vi "Actor Core.vi"(8 "error in (no error)":errorcluster, 11 "Test Interface in":refnum<class "Test Interface.lvclass">) -> (0 "error out":errorcluster, 3 "Actor Framework.lvlib:Actor":refnum<class "Actor.lvclass">)   [LabVIEW 2015, in "Test Interface.lvclass"]
uses:
  Test Interface.lvclass
  <vilib>/ActorFramework/Actor/Actor.lvclass
  Controls/Menu object array.ctl
  Controls/Menu object.ctl
  Test Interface.lvclass/Test Interface.ctl
  <vilib>/ActorFramework/Actor/Actor.lvclass/Actor.ctl
  <vilib>/ActorFramework/Message Enqueuer/Message Enqueuer.lvclass/Message Enqueuer.ctl
  <vilib>/ActorFramework/Message Enqueuer/Init from Existing Queue.vi
  <vilib>/ActorFramework/Message Enqueuer/Enqueue.vi
  <vilib>/ActorFramework/Message Priority Queue/Priority Enqueue.vi
  <vilib>/ActorFramework/Message Enqueuer/Message Enqueuer.lvclass
  <vilib>/ActorFramework/Stop Msg/Stop Msg.lvclass
  Mag Lab Measure Interface/Mag Lab Measure UI.lvclass
panel:
  in  "Menu object array":T1 {"Object name" items=["Select one"]}
  in  "Devices":u16[](array[ring]) items=["dev1", "5051"]
  in  "Stop Button":bool
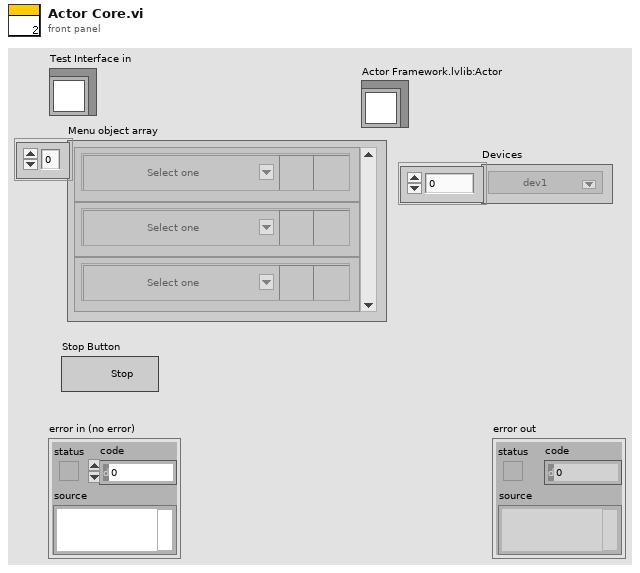
[diagram p1: front panel]
types:
  T1 = typedef "Menu object array.ctl" = T2[]
  T2 = typedef "Menu object.ctl" = cluster{"Object name":u16, "Open parameters":bool, "Remove Button":bool}
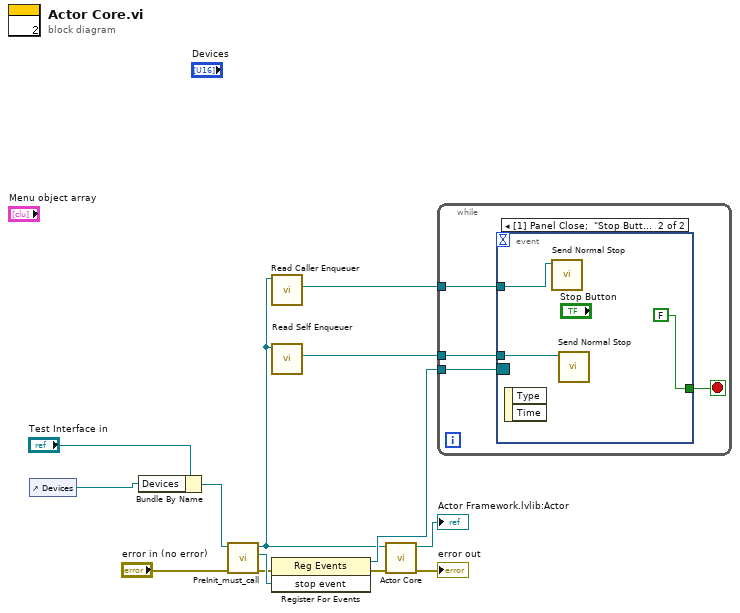
[diagram p0: block diagram]
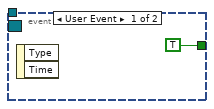
[diagram p2: hidden frame]
diagram:
  n1 = control-ref of="Devices"() -> (w1:refnum<vi>)
  n2 = Bundle By Name(cluster="Test Interface in", "Devices"=w1) -> (w2:refnum<class "Test Interface.lvclass">)
  n3 = call-dynamic "PreInit_must_call.vi"("error in (no error)"="error in (no error)", "Mag Lab Measure Interface in"=w2) -> ("error out"=w5:errorcluster, "stop event"=w11:refnum<user-event>, "Mag Lab Measure Interface out"=w4:refnum<class "Test Interface.lvclass">)  [unwired: 7 in]
  n4 = call <vilib>:"Read Caller Enqueuer.vi"("Actor"=w4) -> ("Caller Enqueuer"=w3:refnum<class "Message Enqueuer.lvclass">)  [unwired: 10 in]
  n5 = call <vilib>:"Read Self Enqueuer.vi"("Actor"=w4) -> ("Self Enqueuer"=w7:refnum<class "Message Enqueuer.lvclass">)  [unwired: 10 in]
  n6 = register-events(error in=w5, w11) -> (reference out=w8:refnum<event-registration>, error out=w9:errorcluster)  [unwired: 1 in]
  n7 = call-parent "Actor Core.vi"("error in (no error)"=w9, "Mag Lab Measure Interface in"=w4) -> ("error out"=→"error out":errorcluster, "Actor Framework.lvlib:Actor"=→"Actor Framework.lvlib:Actor":refnum<class "Actor.lvclass">)  [unwired: 8 in]
  n8 = while {
    tunnel: w8 -> [w17]
    tunnel: w7 -> [w15]
    tunnel: w3 -> [w14]
    stop <- w16 stop-if-true
    n9 = event shown="[1] Panel Close;  \"Stop Button\": Value Change" {
      selector: w17 -> [_ _]
      dyn-events: _ -> [_ _]
      timeout: _ -> [_ _]
      tunnel: [TRUE FALSE] -> w16
      tunnel: w15 -> [_ w20]
      tunnel: w14 -> [_ w19]
      event User Event {
        n10 = event-data() -> ()  [unwired: 1 in, 2 out]
      }
      event Panel Close; "Stop Button": Value Change {
        n11 = event-data() -> ()  [unwired: 1 in, 2 out]
        n12 = call <vilib>:"Send Normal Stop.vi"("Message Enqueuer"=w19) -> ()  [unwired: 10 in, 1 out]
        n13 = call <vilib>:"Send Normal Stop.vi"("Message Enqueuer"=w20) -> ()  [unwired: 10 in, 1 out]
      }
    }
  }
